vi "data_headers_Jan2017.vi"(8 "Experiment Notes":string, 10 "Sample names":T1={"QCM1 sample name"="aQCM2", "QCM2 sample name"="aQCM2", "QCM3 sample name"="aQCM3", "QCM4 sample name"="aQCM4", "QCM5 sample name"="aQCM5", "QCM6 sample name"="aQCM6", "SRS sample name"="sample_SRS", "Keithley 2420 sample name"="Keithley2420", "Keithley 6430 sample name"="Keithley6430", "Keithley 2100 sample name"="Keithley6430", "Gas"="aQCM2", "Vapor"="aQCM2"}) -> (2 "data headers":string[](array[string]))   [LabVIEW 2014]
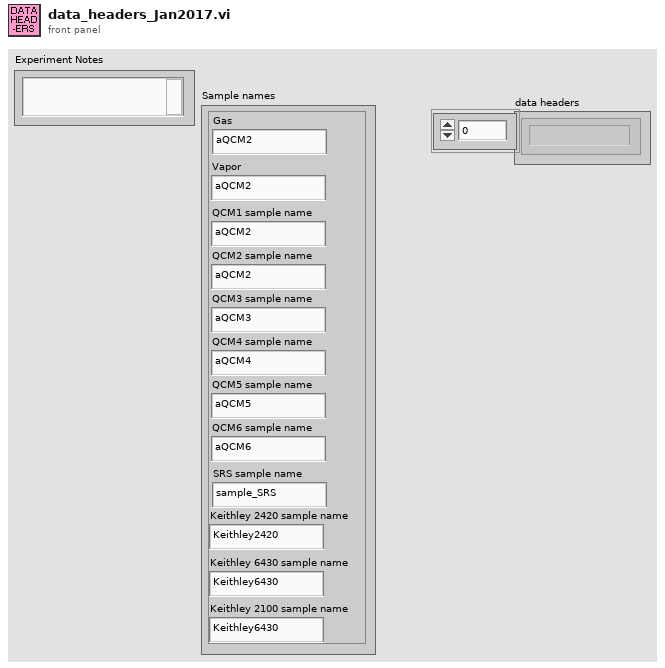
[diagram p1: front panel]
types:
  T1 = cluster{"QCM1 sample name":string, "QCM2 sample name":string, "QCM3 sample name":string, "QCM4 sample name":string, "QCM5 sample name":string, "QCM6 sample name":string, "SRS sample name":string, "Keithley 2420 sample name":string, "Keithley 6430 sample name":string, "Keithley 2100 sample name":string, "Gas":string, "Vapor":string}
  T2 = cluster{string, string, string, string, string, string}
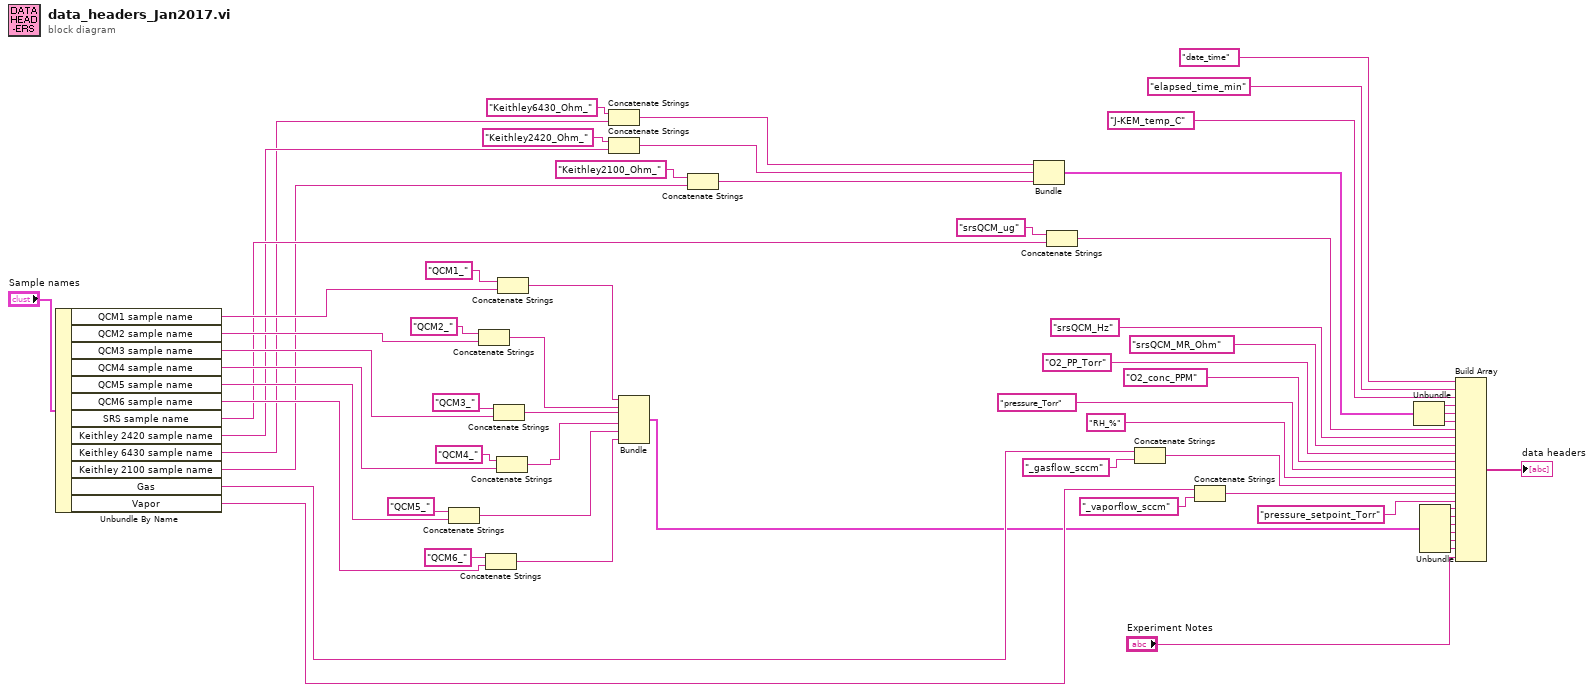
[diagram p0: block diagram]
diagram:
  n1 = Unbundle By Name("Sample names") -> ("QCM1 sample name"=w48:string, "QCM2 sample name"=w45:string, "QCM3 sample name"=w43:string, "QCM4 sample name"=w41:string, "QCM5 sample name"=w38:string, "QCM6 sample name"=w37:string, "SRS sample name"=w34:string, "Keithley 2420 sample name"=w33:string, "Keithley 6430 sample name"=w32:string, "Keithley 2100 sample name"=w30:string, "Gas"=w16:string, "Vapor"=w15:string)
  n2 = Concatenate Strings("QCM5_" ("string"), w38) -> (w9:string)
  n3 = Concatenate Strings("QCM2_" ("string"), w45) -> (w12:string)
  n4 = Concatenate Strings("QCM6_" ("string"), w37) -> (w8:string)
  n5 = Concatenate Strings("QCM3_" ("string"), w43) -> (w11:string)
  n6 = Concatenate Strings("QCM4_" ("string"), w41) -> (w10:string)
  n7 = Concatenate Strings("QCM1_" ("string"), w48) -> (w13:string)
  n8 = Concatenate Strings("Keithley6430_Ohm_", w32) -> (w28:string)
  n9 = Concatenate Strings("Keithley2420_Ohm_" ("element"), w33) -> (w27:string)
  n10 = Bundle(w13, w12, w11, w10, w9, w8) -> (w7:T2)  [unwired: 1 in]
  n11 = Concatenate Strings("Keithley2100_Ohm_" ("element"), w30) -> (w26:string)
  n12 = Bundle(w28, w27, w26) -> (w25:cluster{string, string, string})  [unwired: 1 in]
  n13 = Concatenate Strings("srsQCM_ug", w34) -> (w35:string)
  n14 = Concatenate Strings(w16, "_gasflow_sccm" ("element")) -> (w20:string)
  n15 = Concatenate Strings(w15, "_vaporflow_sccm" ("element")) -> (w19:string)
  n16 = Unbundle(w25) -> (w24:string, w23:string, w22:string)
  n17 = Unbundle(w7) -> (w1:string, w2:string, w3:string, w4:string, w5:string, w6:string)
  n18 = Build Array("date_time", "elapsed_time_min", "J-KEM_temp_C", w24, w23, w22, w35, "srsQCM_Hz", "srsQCM_MR_Ohm", "O2_PP_Torr" ("element"), "O2_conc_PPM" ("element"), "pressure_Torr" ("element"), "RH_%" ("element"), w20, w19, "pressure_setpoint_Torr" ("element"), w1, w2, w3, w4, w5, w6, "Experiment Notes") -> (→"data headers":string[])
